vi "ratometer_beta0.5.vi"() -> ()   [LabVIEW 2021]
uses:
  <vilib>/Utility/error.llb/DialogType.ctl
  0f2237de-6407-6143-a075-b3391785e022.vi
  <vilib>/MakerHub/LINX/Public/Utilities/Open Serial.vi
  <vilib>/MakerHub/LINX/Public/Sensors/Motion/Servo/Servo Open One Channel.vi
  <vilib>/MakerHub/LINX/Public/Sensors/Motion/Servo/Servo Set Pulse Width One Channel.vi
  <vilib>/MakerHub/LINX/Public/Sensors/Motion/Servo/Servo Close One Channel.vi
  <vilib>/Waveform/WDTOps.llb/WDT Waveform Duration DBL.vi
  <vilib>/Waveform/WDTOps.llb/WDT Index Channel DBL.vi
  <vilib>/MakerHub/LINX/LMH-LINX.lvlib
  <vilib>/MakerHub/LINX/Public/Sensors/Motion/Servo/Servo.lvlib
  <vilib>/Utility/TDMS File Viewer/NI_TDMS File Viewer.lvlib
panel:
  in  "Protocol index":dbl
  in  "Reset Controls":bool
  in  "Stop Button":bool
  in  "Tabs":T1(tab)
  in  "Run Protocol":bool
  in  "Trial Parameters":T2={"Condition"="PF", "Angle"=90.0, "Trial Number"=0, "RatID"="K01-XXX", "Side"="R", "Recovery (s)"=45.0} {"Angle" min=30.0 max=150.0 step=10.0}
  out "Recovery Timer (s)":dbl
  in  "Data Directory":path=path "C:/Users/baxterj/Desktop/data"
  in  "Run Trial":bool
  out "Trial - Analog Input":waveform(dbl)[](graph)
  in  "Digitimer Parameters":T3={"Stim Freq (hz)"=100, "Sampling Freq (hz)"=1000, "Stim Duration (ms)"=300, "Padding (ms)"=1000, "Ampltude (mA)"=1.0, "Pulse width\n(microseconds)"=100} {"Stim Duration (ms)" max=1000 step=1; "Stim Freq (hz)" max=20 step=1}
  out "Trigger pulse":waveform(dbl)(graph)
  out "Trial count":u16
  out "Trial Running":bool
  out "TDMS file name":string
  in  "Digitimer Trigger":bool
  out "Trial name":string
  in  "Randomize Protocol":bool
  out "protocol_built":bool
  in  "Trials per angle":u8=3 step=1
  in  "Test Angles (degrees)":dbl[](array[numeric])=[30.0, 50.0, 70.0, 90.0, 110.0, 130.0, 150.0]
  in  "Build Protocol":bool
  out "protocol_array":dbl[][](array[numeric])
  out "randomized order":i32[](array[numeric])
  in  "Serial Port":refnum<visa-resource-name>="N/A"
  in  "Servo Channel":u8=3
  in  "Hardware Parameters":T4={"Servo_gain"=7.18, "Servo_bias"=914.0, "Torque_gain"=119.54, "Torque_bias"=1.99, "Calibration time"=timestamp(3713893022.708219 s since 1904-01-01), "Torque_negate"=0.0} {"Servo_bias" format="%#_13g"; "Servo_gain" format="%#_13g"}
  out "Actual AI Rate":dbl=1000.0 format="%0.2f"
  out "Actual AO Rate":dbl=1000.0 format="%0.2f"
  in  "physical channels":tag="Dev1/ai0:1"
  in  "Analog Trigger":tag="Dev1/ao0"
  in  "TDMS path for Viewer":path
  in  "TDMS Viewer":bool
  in  "Run Trigger":dbl
  in  "Protocol_trigger":dbl
  in  "Wait trigger":dbl
  in  "PWM":u16
  out "n_protocol_trials":i32
  in  "Update name":bool
  out "trigger samples":i32
  # "RATOMETER - VERSION 0.5\n2021-09-04\njoshrbaxter@gmail.com"
  # "Step 1. Set RatID and digitimer notes\nStep 2. If running a protocol, select parameters and 'build' under 'Protocol Builder' tab\nStep 3. Set Digitimer Trigger parameters and click 'update'\nStep 4. Run Single Trial: Move ankle to desired position and click 'Run Trial'\n                                                                     OR\n              Run Protocol: Click 'Run Protocol' and protocol will be completed\n                                      - Protocol can be 'paused' by clicking 'Run Protocol' \n                                      - Protocol can be 'resumed' by clicking 'Run Protocol' when paused\n                                      - Protocol disables 'run' button until protocol is stopped or stops"
  # "CONTROLS"
  # "DIGITIMER"
  # "ARDUINO AND SERVO INITIALIZATION"
  # "DEBUG PANEL\nprogram variables that user SHOULD NOT CHANGE held here for debugging purposes"
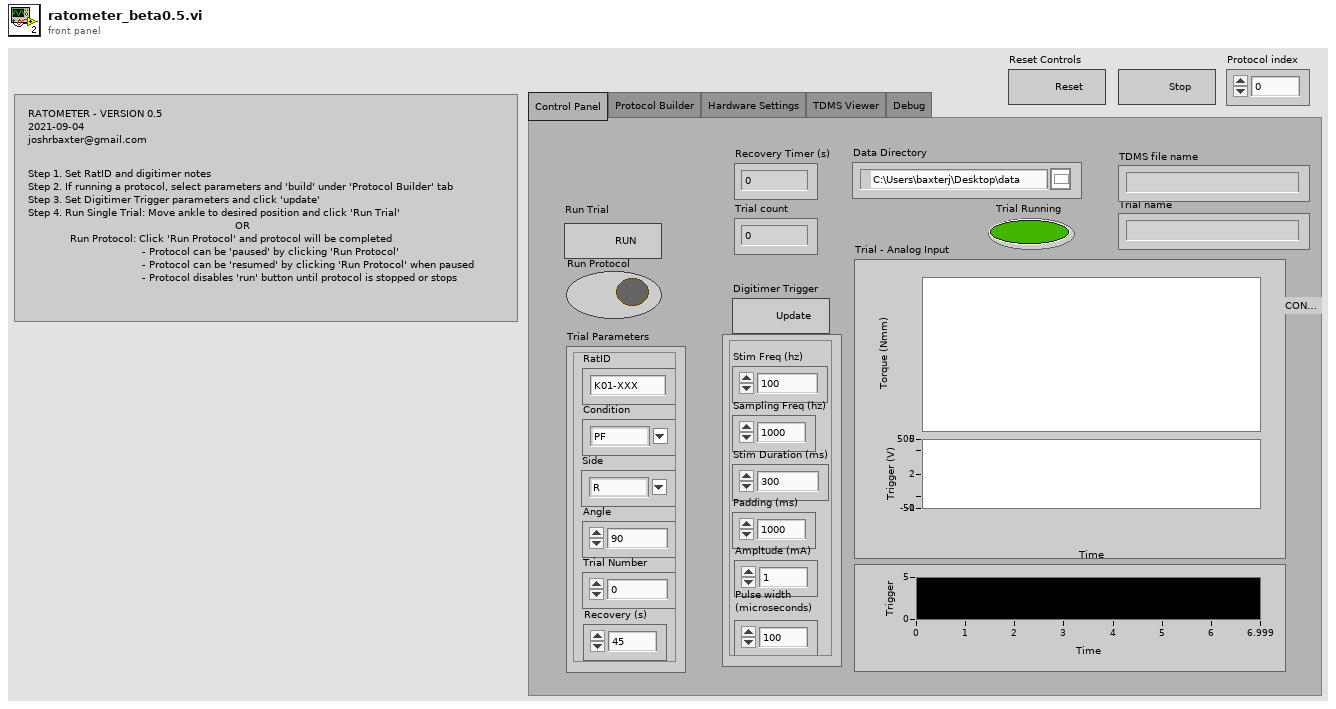
[diagram p1: front panel]
types:
  T1 = enum32{"Control Panel", "Protocol Builder", "Hardware Settings", "TDMS Viewer", "Debug"}
  T2 = cluster{"Condition":string, "Angle":dbl, "Trial Number":u8, "RatID":string, "Side":string, "Recovery (s)":dbl}
  T3 = cluster{"Stim Freq (hz)":u16, "Sampling Freq (hz)":u16, "Stim Duration (ms)":u16, "Padding (ms)":u16, "Ampltude (mA)":dbl, "Pulse width\n(microseconds)":u16}
  T4 = cluster{"Servo_gain":dbl, "Servo_bias":dbl, "Torque_gain":dbl, "Torque_bias":dbl, "Calibration time":timestamp, "Torque_negate":dbl}
  T5 = typedef "DialogType.ctl" = u16
  T6 = typedef "LMH-LINX.lvlib/LINX Ref.ctl" = cluster{"IO":T7, "Interface":T8, "LINX Device Config":T9}
  T7 = typedef "LMH-LINX.lvlib/Platform.ctl" = enum16{"Remote", "Local"}
  T8 = typedef "LMH-LINX.lvlib/Interface.ctl" = enum16{"Serial", "TCP"}
  T9 = typedef "LMH-LINX.lvlib/Device.lvlib/LINX Device Config.ctl" = cluster{"Interface":T8, "COM Port":refnum<visa-resource-name>, "TCP Configuration":T10, "Device Family":u8, "Device ID":u8, "Device Name":string, "TCP Ref":refnum<k5>, "Channels":T11}
  T10 = typedef "LMH-LINX.lvlib/Device.lvlib/TCP Config.ctl" = cluster{"IP Address":string, "Port":u16}
  T11 = typedef "LMH-LINX.lvlib/Channels.ctl" = cluster{"DI":u8[], "DO":u8[], "AI":u8[], "AO":u8[], "PWM":u8[], "QE":u8[], "UART":u8[], "I2C 2":u8[], "SPI":u8[], "CAN":u8[], "Servo":u8[], "AI Ref (V)":dbl, "AI Resolution (Bits)":u8, "AO Ref (V)":dbl, "AO Resolution (Bits)":u8}
  T12 = enum8{"Enabled", "Disabled", "Disabled and Grayed Out"}
  T13 = cluster{"Servo_gain":dbl, "Servo_bias":dbl, "Torque_gain":dbl, "Torque_gain":dbl, "Calibration time":timestamp, "Numeric":dbl}
  T14 = cluster{"Servo_gain":dbl, "Servo_bias":dbl, "Torque_gain":dbl, "Torque_gain":dbl, "Calibration time":timestamp, "Torque_negate":dbl}
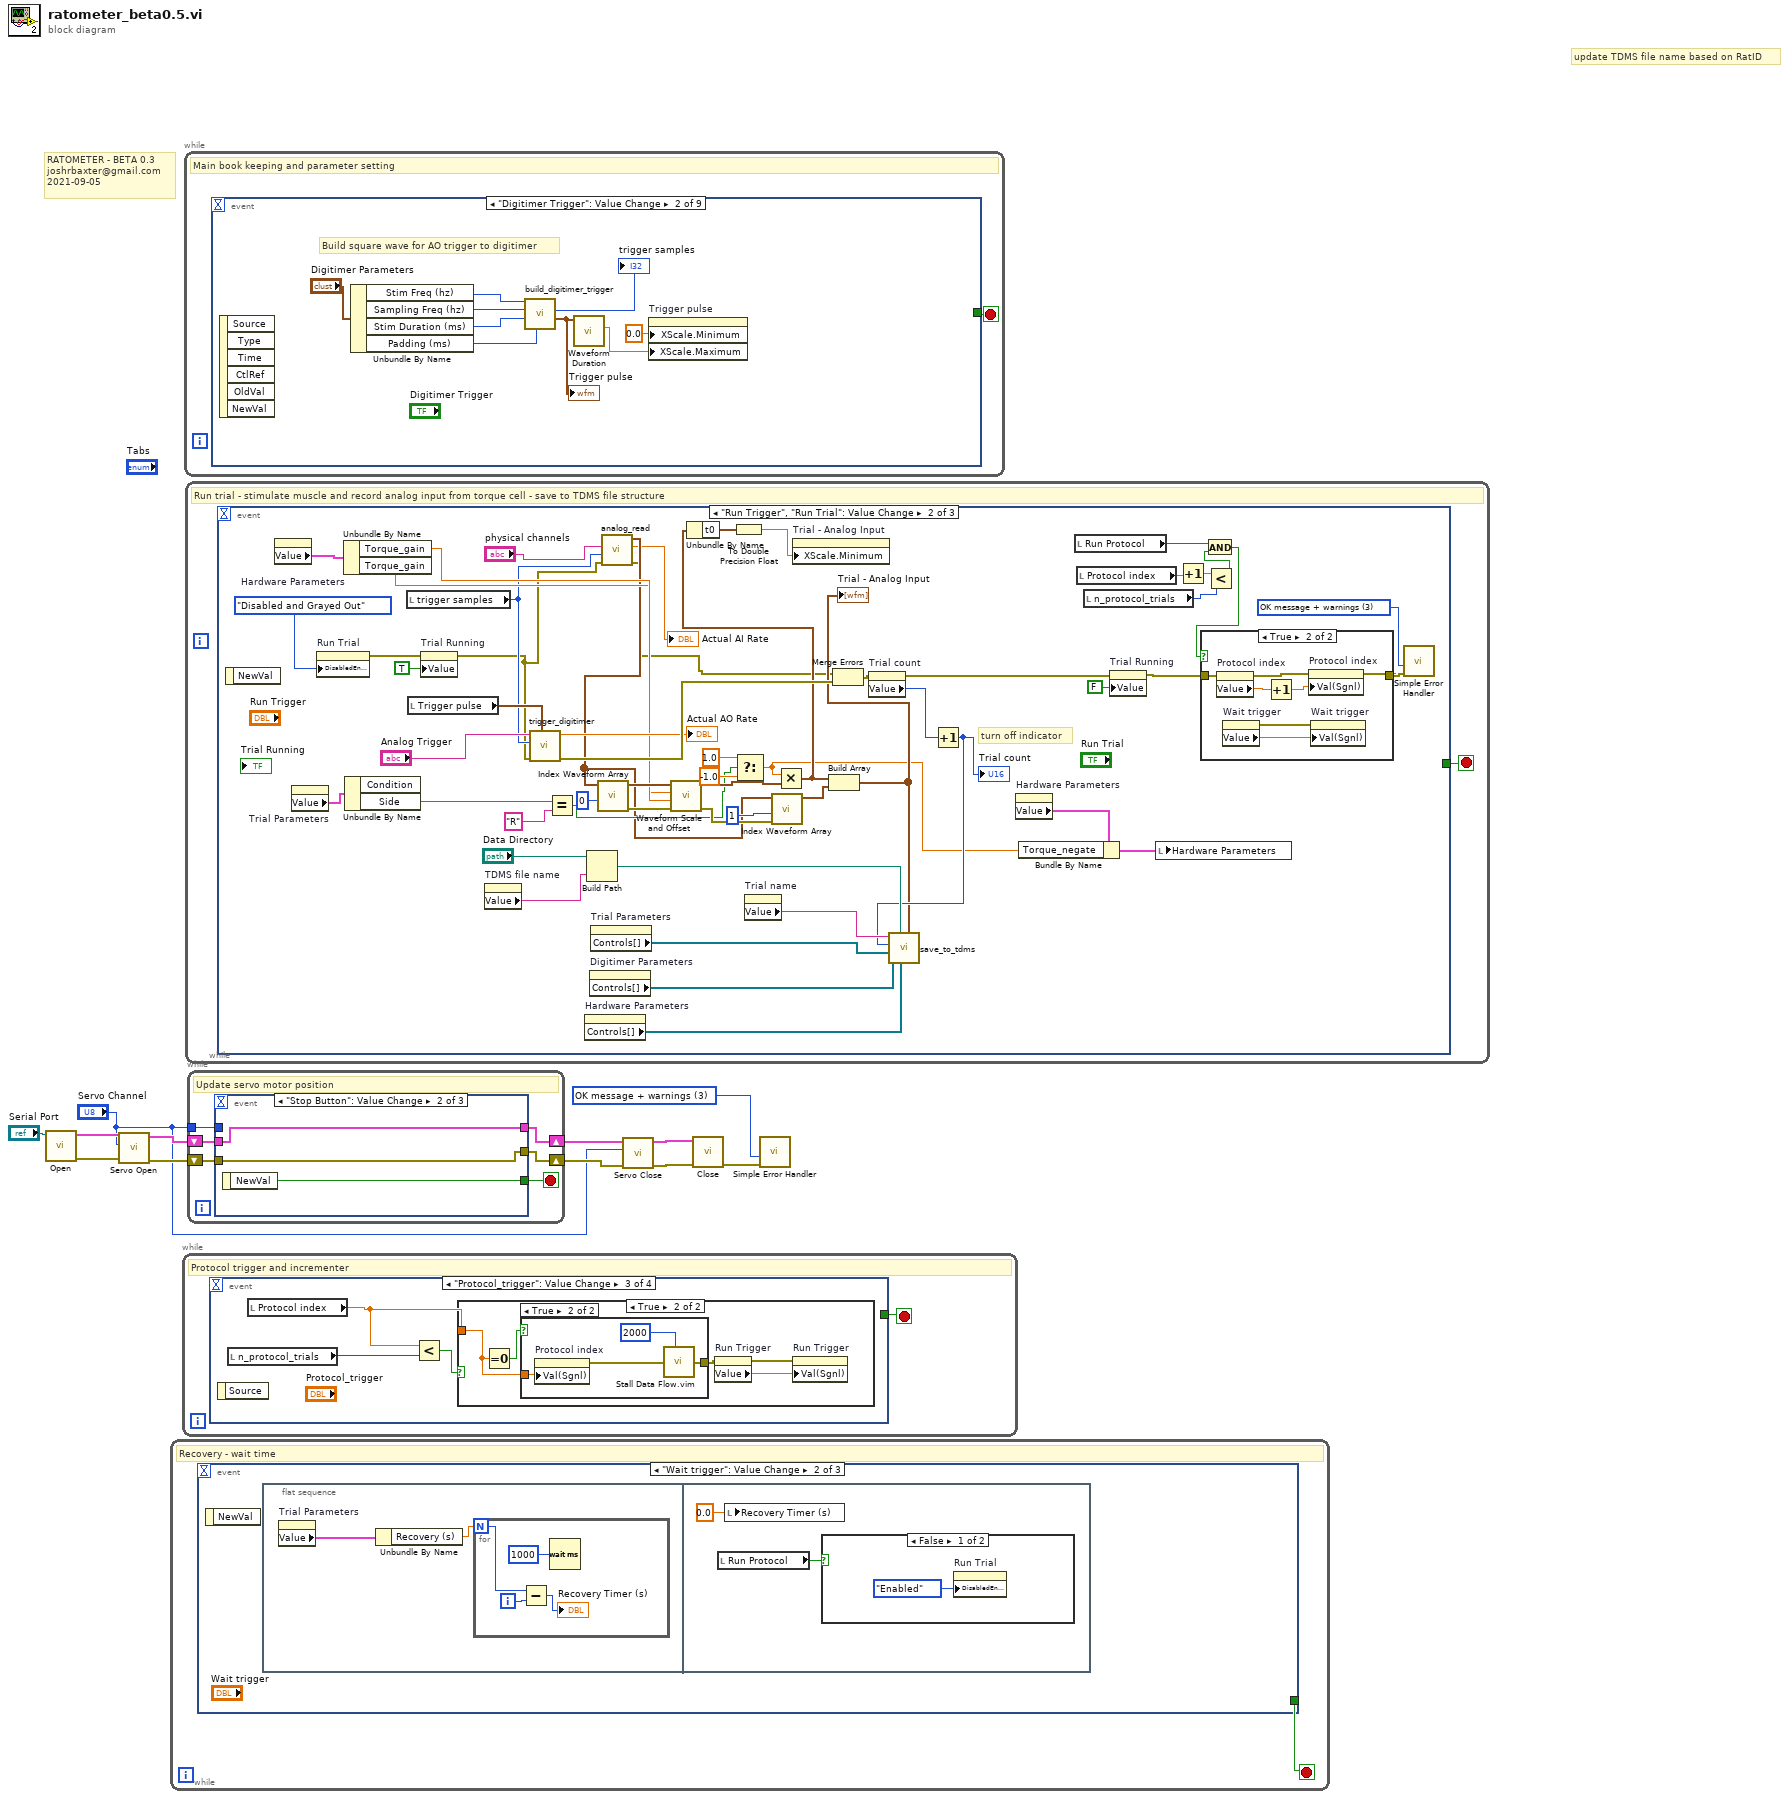
[diagram p0: block diagram]
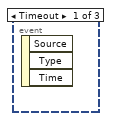
[diagram p2: hidden frame]
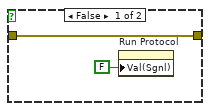
[diagram p3: hidden frame]
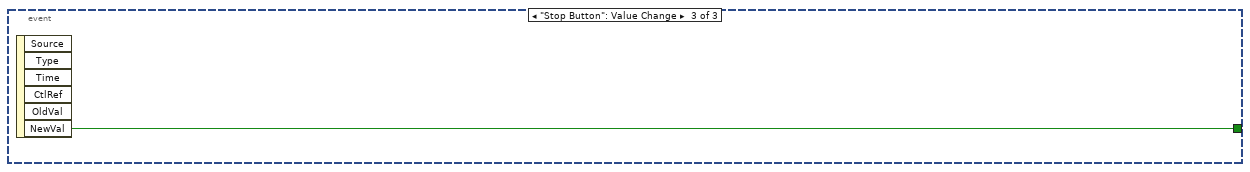
[diagram p4: hidden frame]
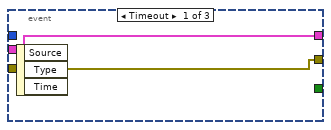
[diagram p5: hidden frame]
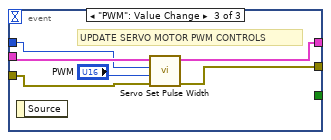
[diagram p6: hidden frame]
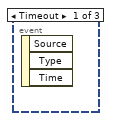
[diagram p7: hidden frame]
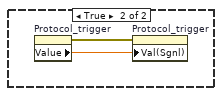
[diagram p8: hidden frame]
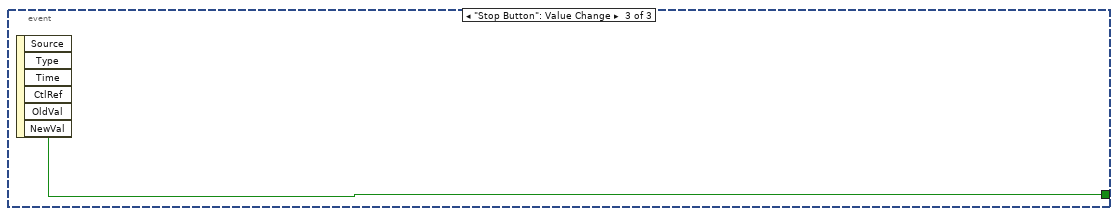
[diagram p9: hidden frame]
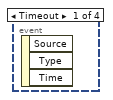
[diagram p10: hidden frame]
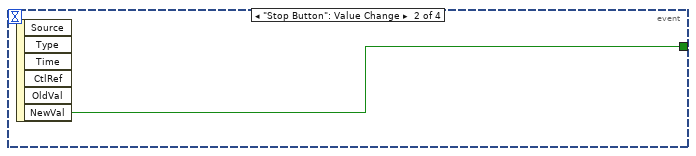
[diagram p11: hidden frame]
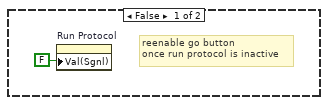
[diagram p12: hidden frame]
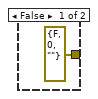
[diagram p13: hidden frame]
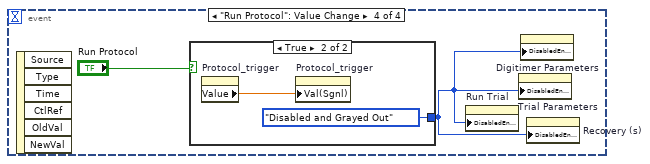
[diagram p14: hidden frame]
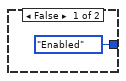
[diagram p15: hidden frame]
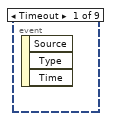
[diagram p16: hidden frame]
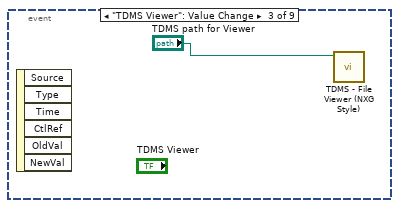
[diagram p17: hidden frame]
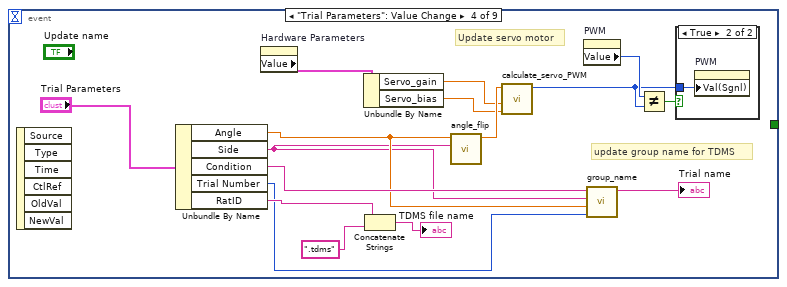
[diagram p18: hidden frame]
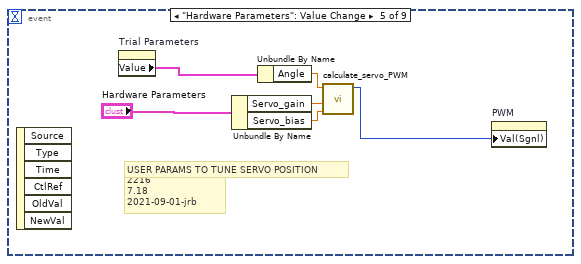
[diagram p20: hidden frame]
diagram:
  w4 = T5 3 items=["no dialog", "OK message", "continue or stop message", "OK message + warnings", "continue/stop + warnings"] ("type of dialog (OK msg:1)")
  # "update TDMS file name based on RatID"
  # "RATOMETER - BETA 0.3\njoshrbaxter@gmail.com\n2021-09-05"
  n1 = call-poly <vilib>:"Open.vi"("Serial Port"="Serial Port") -> ("Error Out"=w10:errorcluster, "LINX Resource"=w12:T6)  [unwired: 8 in, 1 out]
  n2 = call-poly <vilib>:"Servo Open.vi"("Error In"=w10, "Servo Channel"="Servo Channel", "LINX Resource"=w12) -> ("Error Out"=w9:errorcluster, "LINX Resource"=w11:T6)  [unwired: 7 in]
  n3 = while {
    stop <- w13 stop-if-true
    # "Recovery - wait time"
    n4 = event shown="[1] \"Wait trigger\": Value Change" {
      selector: _ -> [_ _ _]
      dyn-events: _ -> [_ _ _]
      timeout: _ -> [_ _ _]
      tunnel: [_ _ w25] -> w13
      event Timeout {
        n5 = event-data() -> ()  [unwired: 1 in, 3 out]
      }
      event "Wait trigger": Value Change {
        n6 = event-data() -> ()  [unwired: 1 in, 1 out]
        n7 = flat-sequence {
          frame #0 {
            n8 = property on="Trial Parameters" class="Clust (strict)"() -> ("Value"=w15:T2)  [unwired: 2 in, 2 out]
            n9 = Unbundle By Name(w15) -> ("Recovery (s)"=w14:dbl)
            n10 = for {
              N: w14 -> [w19]
              i -> [w18]
              n11 = Subtract(x=w19, y=w18) -> (x-y=→"Recovery Timer (s)":i32)
              n12 = Wait (ms)(milliseconds to wait=u32 1000) -> ()  [unwired: 1 out]
            }
          }
          frame #1 {
            n13 = local read "Run Protocol"() -> (w20:bool)
            n14 = local write "Recovery Timer (s)"(0.0 ("Recovery Timer (s)")) -> ()
            n15 = case shown="False" w20 {
              frame False {
                n16 = property on="Run Trial" class="Bool"("DisabledEnum"=T12."Enabled" ("Disabled")) -> ()  [unwired: 2 in, 2 out]
              }
              frame True {
                n17 = property on="Protocol_trigger" class="DigNum (strict)"() -> (error out=w24:errorcluster, "Value"=w23:dbl)  [unwired: 2 in, 1 out]
                n18 = property on="Protocol_trigger" class="DigNum (strict)"(error in=w24, "Val(Sgnl)"=w23) -> ()  [unwired: 1 in, 2 out]
              }
            }
          }
        }
      }
      event "Stop Button": Value Change {
        n19 = event-data() -> ("NewVal"=w25:bool)  [unwired: 1 in, 5 out]
      }
    }
  }
  n20 = while {
    stop <- w26 stop-if-true
    # "Protocol trigger and incrementer"
    n21 = event shown="[2] \"Protocol_trigger\": Value Change" {
      selector: _ -> [_ _ _ _]
      dyn-events: _ -> [_ _ _ _]
      timeout: _ -> [_ _ _ _]
      tunnel: [_ w27 _ _] -> w26
      event Timeout {
        n22 = event-data() -> ()  [unwired: 1 in, 3 out]
      }
      event "Stop Button": Value Change {
        n23 = event-data() -> ("NewVal"=w27:bool)  [unwired: 1 in, 5 out]
      }
      event "Protocol_trigger": Value Change {
        n24 = event-data() -> ()  [unwired: 1 in, 1 out]
        n25 = local read "n_protocol_trials"() -> (w30:i32)
        n26 = local read "Protocol index"() -> (w28:dbl)
        n27 = Less?(x=w28, y=w30) -> (x < y?=w29:bool)
        n28 = case shown="True" w29 {
          tunnel: w28 -> [_ w32]
          frame False {
            # "reenable go button\nonce run protocol is inactive"
            n29 = property on="Run Protocol" class="Bool (strict)"("Val(Sgnl)"=FALSE ("Run Protocol")) -> ()  [unwired: 2 in, 2 out]
          }
          frame True {
            n30 = Equal To 0?(x=w32) -> (x = 0?=w34:bool)
            n31 = case shown="True" w34 {
              tunnel: [errorcluster {"status"=FALSE, "code"=0, "source"=""} ("error out") w39] -> w33
              tunnel: w32 -> [_ w41]
              frame False {
              }
              frame True {
                n32 = property on="Protocol index" class="DigNum (strict)"("Val(Sgnl)"=w41) -> (error out=w40:errorcluster)  [unwired: 2 in, 1 out]
                n33 = call "Stall Data Flow.vim"("value in"=w40, "milliseconds to wait"=u32 2000) -> ("value out"=w39:errorcluster)  [unwired: 1 out]
              }
            }
            n34 = property on="Run Trigger" class="DigNum (strict)"(error in=w33) -> (error out=w36:errorcluster, "Value"=w35:dbl)  [unwired: 1 in, 1 out]
            n35 = property on="Run Trigger" class="DigNum (strict)"(error in=w36, "Val(Sgnl)"=w35) -> ()  [unwired: 1 in, 2 out]
          }
        }
      }
      event "Run Protocol": Value Change {
        n36 = event-data() -> ()  [unwired: 1 in, 6 out]
        n37 = case shown="True" "Run Protocol" {
          tunnel: [T12."Enabled" ("Disabled") T12."Disabled and Grayed Out" ("Disabled")] -> w43
          frame False {
          }
          frame True {
            n38 = property on="Protocol_trigger" class="DigNum (strict)"() -> ("Value"=w46:dbl)  [unwired: 2 in, 2 out]
            n39 = property on="Protocol_trigger" class="DigNum (strict)"("Val(Sgnl)"=w46) -> ()  [unwired: 2 in, 2 out]
          }
        }
        n40 = property on="Run Trial" class="Bool"("DisabledEnum"=w43) -> ()  [unwired: 2 in, 2 out]
        n41 = property on="Trial Parameters" class="Clust (strict)"("DisabledEnum"=w43) -> ()  [unwired: 2 in, 2 out]
        n42 = property on="Digitimer Parameters" class="Clust (strict)"("DisabledEnum"=w43) -> ()  [unwired: 2 in, 2 out]
        n43 = property on="Recovery (s)" class="DigNum (strict)"("DisabledEnum"=w43) -> ()  [unwired: 2 in, 2 out]
      }
    }
  }
  n44 = while {
    stop <- w47 stop-if-true
    # "Main book keeping and parameter setting"
    n45 = event shown="[1] \"Digitimer Trigger\": Value Change" {
      selector: _ -> [_ _ _ _ _ _ _ _ _]
      dyn-events: _ -> [_ _ _ _ _ _ _ _ _]
      timeout: _ -> [_ _ _ _ _ _ _ _ _]
      tunnel: [_ _ _ _ _ _ _ _ "Stop Button"] -> w47
      event Timeout {
        n46 = event-data() -> ()  [unwired: 1 in, 3 out]
      }
      event "Digitimer Trigger": Value Change {
        # "Build square wave for AO trigger to digitimer"
        n47 = event-data() -> ()  [unwired: 1 in, 6 out]
        n48 = Unbundle By Name("Digitimer Parameters") -> ("Stim Freq (hz)"=w52:u16, "Sampling Freq (hz)"=w51:u16, "Stim Duration (ms)"=w50:u16, "Padding (ms)"=w49:u16)
        n49 = call "build_digitimer_trigger.vi"("Padding (ms)"=w49, "Stim Duration (ms)"=w50, "Sampling Freq (hz)"=w51, "Stim Freq (hz)"=w52) -> ("waveform out"=w56:waveform(dbl), "number of samples"=→"trigger samples":i32)  [unwired: 5 in, 1 out]
        "Trigger pulse" <- w56
        n50 = call-poly <vilib>:"Waveform Duration.vi"("waveform in"=w56) -> ("duration"=w54:dbl)  [unwired: 8 in, 2 out]
        n51 = property on="Trigger pulse" class="WFGraph (strict)"("XScale.Minimum"=0.0 ("X Scale.Range:Minimum"), "XScale.Maximum"=w54) -> ()  [unwired: 2 in, 2 out]
      }
      event "TDMS Viewer": Value Change {
        n52 = event-data() -> ()  [unwired: 1 in, 6 out]
        n53 = call <vilib>:"TDMS - File Viewer (NXG Style).vi"("file in"="TDMS path for Viewer") -> ()  [unwired: 9 in, 2 out]
      }
      event "Trial Parameters": Value Change {
        # "update group name for TDMS"
        # "Update servo motor"
        n54 = event-data() -> ()  [unwired: 1 in, 6 out]
        n55 = Unbundle By Name("Trial Parameters") -> ("Angle"=w61:dbl, "Side"=w59:string, "Condition"=w66:string, "Trial Number"=w60:u8, "RatID"=w67:string)
        n56 = property on="Hardware Parameters" class="Clust (strict)"() -> ("Value"=w64:T13)  [unwired: 2 in, 2 out]
        n57 = Unbundle By Name(w64) -> ("Servo_gain"=w63:dbl, "Servo_bias"=w62:dbl)
        n58 = Concatenate Strings(w67, ".tdms" ("string")) -> (→"TDMS file name":string)
        n59 = call "angle_flip.vi"("Side in"=w59, "Angle in"=w61) -> ("Angle out"=w69:dbl)  [unwired: 8 in, 1 out]
        n60 = call "calculate_servo_PWM.vi"("Angle"=w69, "Servo_gain"=w63, "Servo_bias"=w62) -> ("Numeric"=w71:u16)  [unwired: 7 in]
        n61 = property on="PWM" class="DigNum (strict)"() -> ("Value"=w73:u16)  [unwired: 2 in, 2 out]
        n62 = call "group_name.vi"("Condition"=w66, "Side"=w59, "Angle"=w61, "Trial num"=w60) -> ("Trial name"=→"Trial name":string)  [unwired: 6 in]
        n63 = Not Equal?(x=w73, y=w71) -> (x != y?=w72:bool)
        n64 = case shown="True" w72 {
          tunnel: w71 -> [_ w74]
          frame False {
          }
          frame True {
            n65 = property on="PWM" class="DigNum (strict)"("Val(Sgnl)"=w74) -> ()  [unwired: 2 in, 2 out]
          }
        }
      }
      event "Hardware Parameters": Value Change {
        # "914\n2216\n7.18\n2021-09-01-jrb"
        # "USER PARAMS TO TUNE SERVO POSITION"
        n66 = event-data() -> ()  [unwired: 1 in, 6 out]
        n67 = property on="Trial Parameters" class="Clust (strict)"() -> ("Value"=w80:T2)  [unwired: 2 in, 2 out]
        n68 = Unbundle By Name("Hardware Parameters") -> ("Servo_gain"=w76:dbl, "Servo_bias"=w75:dbl)
        n69 = Unbundle By Name(w80) -> ("Angle"=w79:dbl)
        n70 = call "calculate_servo_PWM.vi"("Angle"=w79, "Servo_gain"=w76, "Servo_bias"=w75) -> ("Numeric"=w78:u16)  [unwired: 7 in]
        n71 = property on="PWM" class="DigNum (strict)"("Val(Sgnl)"=w78) -> ()  [unwired: 2 in, 2 out]
      }
      event "Reset Controls": Value Change {
        w81 = 0.0 ("Protocol count")
        n72 = event-data() -> ()  [unwired: 1 in, 6 out]
        n73 = local write "Protocol index"(w81) -> ()
        n74 = local write "Protocol_trigger"(w81) -> ()
        n75 = local write "Recovery Timer (s)"(w81) -> ()
        n76 = local write "Trial count"(w81) -> ()
      }
      event "Protocol index": Value Change {
        # "Run guided protocol"
        # "When driver loop increments 'protocol count' - update trial info"
        n77 = event-data() -> ()  [unwired: 1 in, 6 out]
        n78 = case shown="True" "Randomize Protocol" {
          tunnel: "Protocol index" -> [w93 w95]
          tunnel: [w93 w94] -> w92
          frame False {
          }
          frame True {
            n79 = local read "randomized order"() -> (w96:i32[])
            n80 = Index Array(array=w96, index=w95) -> (element=w94:i32)
          }
        }
        n81 = local read "protocol_array"() -> (w88:dbl[][])
        n82 = Index Array(array=w88, index (row)=w92) -> (element=w89:dbl[])  [unwired: 1 in]
        n83 = property on="Trial Parameters" class="Clust (strict)"() -> ("Value"=w85:T2)  [unwired: 2 in, 2 out]
        n84 = Index Array(array=w89, index=0) -> (element=w83:dbl)
        n85 = Index Array(array=w89, index=1) -> (element=w82:dbl)
        n86 = Bundle By Name(cluster=w85, "Trial Number"=w83, "Angle"=w82) -> (w84:T2)
        n87 = property on="Trial Parameters" class="Clust (strict)"("Val(Sgnl)"=w84) -> ()  [unwired: 2 in, 2 out]
      }
      event "Build Protocol": Value Change {
        # "Build 2D array with trial numbers and ankle angles for guided protocol"
        n88 = event-data() -> ()  [unwired: 1 in, 6 out]
        n89 = call "build_protocol.vi"("Test Angles (degrees)"="Test Angles (degrees)", "Trials per angle"="Trials per angle") -> ("shuffled array"=→"randomized order":i32[], "Numeric"=→"n_protocol_trials":i32, "Array"=→"protocol_array":dbl[][])  [unwired: 7 in]
        "protocol_built" <- TRUE ("protocol_built")
      }
      event "Stop Button": Value Change {
        n90 = event-data() -> ()  [unwired: 1 in, 6 out]
      }
    }
  }
  n91 = while {
    stop <- w104 stop-if-true
    # "Run trial - stimulate muscle and record analog input from torque cell - save to TDMS file structure"
    n92 = event shown="[1] \"Run Trigger\", \"Run Trial\": Value Change" {
      selector: _ -> [_ _ _]
      dyn-events: _ -> [_ _ _]
      timeout: _ -> [_ _ _]
      tunnel: [_ _ w171] -> w104
      event Timeout {
        n93 = event-data() -> ()  [unwired: 1 in, 3 out]
      }
      event "Run Trigger", "Run Trial": Value Change {
        w156 = T5 3 items=["no dialog", "OK message", "continue or stop message", "OK message + warnings", "continue/stop + warnings"] ("type of dialog (OK msg:1)")
        # "turn off indicator"
        n94 = event-data() -> ()  [unwired: 1 in, 1 out]
        n95 = property on="Hardware Parameters" class="Clust (strict)"() -> ("Value"=w142:T13)  [unwired: 2 in, 2 out]
        n96 = property on="Trial Parameters" class="Clust (strict)"() -> ("Value"=w124:T2)  [unwired: 2 in, 2 out]
        n97 = property on="Run Trial" class="Bool"("DisabledEnum"=T12."Disabled and Grayed Out" ("Disabled")) -> (error out=w158:errorcluster)  [unwired: 2 in, 1 out]
        n98 = Unbundle By Name(w142) -> ("Torque_gain"=w129:dbl, "Torque_gain"=w128:dbl)
        n99 = Unbundle By Name(w124) -> ("Side"=w119:string)  [unwired: 1 out]
        n100 = local read "trigger samples"() -> (w110:i32)
        n101 = local read "Trigger pulse"() -> (w144:waveform(dbl))
        n102 = property on="Trial Running" class="Bool (strict)"(error in=w158, "Value"=TRUE ("Boolean")) -> (error out=w109:errorcluster)  [unwired: 1 in, 1 out]
        n103 = property on="TDMS file name" class="Str"() -> ("Value"=w140:string)  [unwired: 2 in, 2 out]
        n104 = call "trigger_digitimer.vi"("data"=w144, "error in"=w109, "trigger samples"=w110, "physical channels"="Analog Trigger") -> ("error out"=w154:errorcluster, "SampClk.Rate"=→"Actual AO Rate":dbl)  [unwired: 6 in]
        n105 = Equal?(x=w119, y="R") -> (x = y?=w117:bool)
        n106 = property on="Hardware Parameters" class="Clust (strict)"() -> ("Controls[]"=w134:refnum<vi>[])  [unwired: 2 in, 2 out]
        n107 = Build Path(base path="Data Directory", name or relative path=w140) -> (appended path=w138:path)
        n108 = property on="Digitimer Parameters" class="Clust (strict)"() -> ("Controls[]"=w135:refnum<vi>[])  [unwired: 2 in, 2 out]
        n109 = property on="Trial Parameters" class="Clust (strict)"() -> ("Controls[]"=w136:refnum<vi>[])  [unwired: 2 in, 2 out]
        n110 = call "analog_read.vi"("physical channels"="physical channels", "samples per channel"=w110, "error in"=w109) -> ("data"=w108:waveform(dbl)[], "Actual AI Rate"=→"Actual AI Rate":dbl, "error out"=w106:errorcluster)  [unwired: 5 in]
        n111 = call-poly <vilib>:"Index Waveform Array.vi"("index"=0, "waveform array"=w108) -> ("error out"=w131:errorcluster, "waveform"=w130:waveform(dbl))  [unwired: 8 in]
        n112 = call <vilib>:"Waveform Scale and Offset.vi"("error in (no error)"=w131, "scale"=w129, "offset"=w128, "waveform in"=w130) -> ("error out"=w122:errorcluster, "waveform out"=w125:waveform(dbl))  [unwired: 6 in]
        n113 = Select(t=1.0, s=w117, f=-1.0) -> (s? t:f=w112:dbl)
        n114 = property on="Trial name" class="Str"() -> ("Value"=w137:string)  [unwired: 2 in, 2 out]
        n115 = call-poly <vilib>:"Index Waveform Array.vi"("error in (no error)"=w122, "index"=1, "waveform array"=w108) -> ("waveform"=w121:waveform(dbl))  [unwired: 7 in, 1 out]
        n116 = Multiply(x=w112, y=w125) -> (x*y=w116:waveform(dbl))
        n117 = Unbundle By Name(w116) -> ("t0"=w115:timestamp)
        n118 = To Double Precision Float(number=w115) -> (double precision float=w152:dbl)
        n119 = property on="Trial - Analog Input" class="WFChart (strict)"("XScale.Minimum"=w152) -> ()  [unwired: 2 in, 2 out]
        n120 = Build Array(w116, w121) -> (w120:waveform(dbl)[])
        "Trial - Analog Input" <- w120
        n121 = Merge Errors(w106, w154) -> (w151:errorcluster)
        n122 = property on="Trial count" class="DigNum (strict)"(error in=w151) -> (error out=w105:errorcluster, "Value"=w139:u16)  [unwired: 1 in, 1 out]
        n123 = Increment(x=w139) -> (x+1=w133:u16)
        "Trial count" <- w133
        n124 = call "save_to_tdms.vi"("data"=w120, "Hardware params"=w134, "file path"=w138, "Digitimer params"=w135, "Trial params"=w136, "Trial Count"=w133, "Group name"=w137) -> ()  [unwired: 5 in]
        n125 = property on="Hardware Parameters" class="Clust (strict)"() -> ("Value"=w113:T14)  [unwired: 2 in, 2 out]
        n126 = Bundle By Name(cluster=w113, "Torque_negate"=w112) -> (w114:T14)
        n127 = local read "Run Protocol"() -> (w146:bool)
        n128 = local read "Protocol index"() -> (w148:dbl)
        n129 = local read "n_protocol_trials"() -> (w149:i32)
        n130 = property on="Trial Running" class="Bool (strict)"(error in=w105, "Value"=FALSE ("Boolean")) -> (error out=w157:errorcluster)  [unwired: 1 in, 1 out]
        n131 = local write "Hardware Parameters"(w114) -> ()
        n132 = Increment(x=w148) -> (x+1=w147:dbl)
        n133 = Less?(x=w147, y=w149) -> (x < y?=w150:bool)
        n134 = And(x=w146, y=w150) -> (x .and. y?=w145:bool)
        n135 = case shown="True" w145 {
          tunnel: w157 -> [w163 w167]
          tunnel: [w163 w166] -> w155
          frame False {
            n136 = property on="Run Protocol" class="Bool (strict)"("Val(Sgnl)"=FALSE ("Value (Signaling)")) -> ()  [unwired: 2 in, 2 out]
          }
          frame True {
            n137 = property on="Protocol index" class="DigNum (strict)"(error in=w167) -> (error out=w168:errorcluster, "Value"=w170:dbl)  [unwired: 1 in, 1 out]
            n138 = property on="Wait trigger" class="DigNum (strict)"() -> (error out=w165:errorcluster, "Value"=w164:dbl)  [unwired: 2 in, 1 out]
            n139 = Increment(x=w170) -> (x+1=w169:dbl)
            n140 = property on="Protocol index" class="DigNum (strict)"(error in=w168, "Val(Sgnl)"=w169) -> (error out=w166:errorcluster)  [unwired: 1 in, 1 out]
            n141 = property on="Wait trigger" class="DigNum (strict)"(error in=w165, "Val(Sgnl)"=w164) -> ()  [unwired: 1 in, 2 out]
          }
        }
        n142 = call <vilib>:"Simple Error Handler.vi"("type of dialog (OK msg:1)"=w156, "error in (no error)"=w155) -> ()  [unwired: 3 in, 5 out]
      }
      event "Stop Button": Value Change {
        n143 = event-data() -> ("NewVal"=w171:bool)  [unwired: 1 in, 5 out]
      }
    }
  }
  n144 = while {
    shift-right: [w174] -> w3
    shift-left: w11 -> [w176]
    shift-right: [w173] -> w2
    shift-left: w9 -> [w175]
    tunnel: "Servo Channel" -> [w172]
    stop <- w177 stop-if-true
    # "Update servo motor position"
    n145 = event shown="[1] \"Stop Button\": Value Change" {
      selector: _ -> [_ _ _]
      dyn-events: _ -> [_ _ _]
      timeout: _ -> [_ _ _]
      tunnel: [_ w182 _] -> w177
      tunnel: w176 -> [w179 w181 w188]
      tunnel: w175 -> [w178 w180 w187]
      tunnel: [w178 w180 w186] -> w173
      tunnel: [w179 w181 w185] -> w174
      tunnel: w172 -> [_ _ w183]
      event Timeout {
        n146 = event-data() -> ()  [unwired: 1 in, 3 out]
      }
      event "Stop Button": Value Change {
        n147 = event-data() -> ("NewVal"=w182:bool)  [unwired: 1 in]
      }
      event "PWM": Value Change {
        # "UPDATE SERVO MOTOR PWM CONTROLS"
        n148 = event-data() -> ()  [unwired: 1 in, 1 out]
        n149 = call-poly <vilib>:"Servo Set Pulse Width.vi"("Error In"=w187, "Pulse Width (uS)"="PWM", "Servo Channel"=w183, "LINX Resource"=w188) -> ("Error Out"=w186:errorcluster, "LINX Resource"=w185:T6)  [unwired: 6 in]
      }
    }
  }
  n150 = call-poly <vilib>:"Servo Close.vi"("Error In"=w2, "Servo Channel"="Servo Channel", "LINX Resource"=w3) -> ("Error Out"=w8:errorcluster, "LINX Resource"=w7:T6)  [unwired: 7 in]
  n151 = call <vilib>:"Close.vi"("Error In"=w8, "LINX Resource"=w7) -> ("Error Out"=w5:errorcluster)  [unwired: 9 in]
  n152 = call <vilib>:"Simple Error Handler.vi"("type of dialog (OK msg:1)"=w4, "error in (no error)"=w5) -> ()  [unwired: 3 in, 5 out]
